vi "Read Setpoint.vi"(8 "error in (no error)":errorcluster, 11 "VISA resource name":refnum<visa-resource-name>) -> (0 "error out":errorcluster, 2 "Setpoint Info Out":T1={"Number"=0, "Enable"=FALSE, "Temperature"=0.0, "Window"=2.0, "Soak Time"=60, "Ramp Rate"=9999.0} {"Ramp Rate" min=0.0 max=9999.0 step=1.0 format="%#.1f"; "Soak Time" min=0 max=9999 step=1 format="%#.0f"; "Window" min=0.1 max=9.9 step=0.1 format="%.1f"; "Temperature" min=-150.0 max=225.0 step=0.1 format="%.1f"; "Number" min=0 max=17}, 3 "VISA resource name out":refnum<visa-resource-name>)   [LabVIEW 2012, in "Temptronic TP04300.lvlib"]
doc: "This VI allows to querry the setpoint parameters, such as\n\n<b>Setpoint Number</b>, for either control or configuration\nValid range: 0-17 - for the Cycle Screen\n 0-2 - for the Operator Screen\n \n<b>Setpoint Enable/disable</b> from the cycle list.\nFalse - disable setpoint\nTrue - enable setpoint\n\n<b>Setpoint temperature</b>\nValid Range: \n -150.0 to 225.0 in the Cycle Screen for any setpoint\n 25.0 to 225.0 for setpoint #0 in Operator Screen\n 15.0 to 35.0 for setpoint #1 in Operator Screen\n -150.0 to 25.0 for setpoint #2 in Operator Screen\n\nNote: Entering a value greater than maximum air temperature limit or\nless than minimum air temperature limit will cause \"out of range error\" \n\n\n<b>Setpoint temperature window</b>\nValid Range: 0.1 to 9.9 \n\nNote: The window is the maximum positive or negative deviation from \nthe temperature setpoint allowable for an \"at temperature\" condition. \n\n<b>Setpoint the soak time</b>\nValid Range: 0 to 9999\n\n<b>Setpoint ramp rate</b>\nValid Range: 0 to 99.9 with 0.1C temperature resolution\n or 100 to 9999 with 1C temperature resolution"
uses:
  <instrlib>/Temptronic TP04300/Temptronic TP04300.lvlib
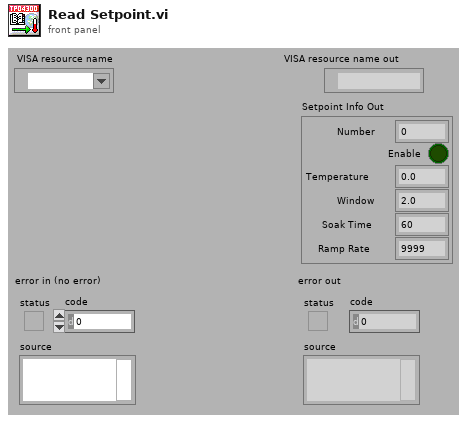
[diagram p1: front panel]
types:
  T1 = cluster{"Number":i32, "Enable":bool, "Temperature":dbl, "Window":dbl, "Soak Time":i32, "Ramp Rate":dbl}
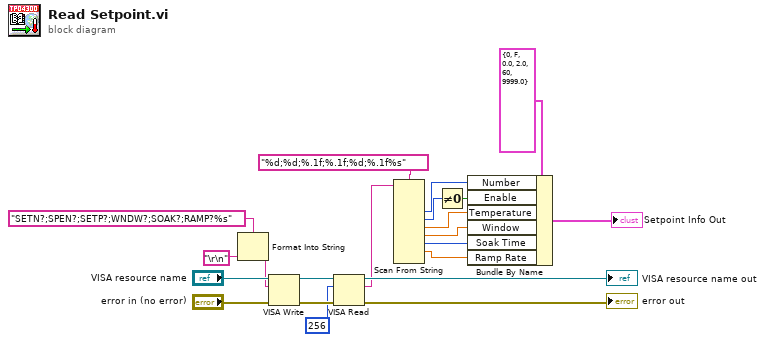
[diagram p0: block diagram]
diagram:
  n1 = Format Into String(format string="SETN?;SPEN?;SETP?;WNDW?;SOAK?;RAMP?%s" ("multi-line string"), "\r\n") -> (resulting string=w19:string)  [unwired: 2 in, 1 out]
  n2 = VISA Write(VISA resource name="VISA resource name", write buffer=w19, error in (no error)="error in (no error)") -> (VISA resource name out=w12:refnum<visa-resource-name>, error out=w14:errorcluster)  [unwired: 1 out]
  n3 = VISA Read(VISA resource name=w12, byte count=u32 256, error in (no error)=w14) -> (VISA resource name out=→"VISA resource name out":refnum<visa-resource-name>, read buffer=w1:string, error out=→"error out":errorcluster)  [unwired: 1 out]
  n4 = Scan From String(format string="%d;%d;%.1f;%.1f;%d;%.1f%s" ("multi-line string"), input string=w1) -> (output 1=w8:i32, output 2=w7:i32, output 3=w5:dbl, output 4=w4:dbl, output 5=w3:i32, output 6=w2:dbl)  [unwired: 10 in, 3 out]
  n5 = Not Equal To 0?(x=w7) -> (x != 0?=w6:bool)
  n6 = Bundle By Name(cluster=T1 {"Number"=0, "Enable"=FALSE, "Temperature"=0.0, "Window"=2.0, "Soak Time"=60, "Ramp Rate"=9999.0} ("Setpoint Info"), "Number"=w8, "Enable"=w6, "Temperature"=w5, "Window"=w4, "Soak Time"=w3, "Ramp Rate"=w2) -> (→"Setpoint Info Out":T1)
